vi "ADC Get Current Setup.vi"(8 "error in":errorcluster, 11 "adc session in":T12={"niScope"={"channel cfg"=[], "sessions"=[], "multi cards"=FALSE, "channels"=0, "type"=enum."n/a", "memory [B/chn]"=0, "ext. clock [Hz]"=0.0, "samples count"=0, "use streaming"=FALSE, "proc setup"={"packet size [smpl]"=0, "current timeout [s]"=0.0, "blk2blk timeout [s]"=0.0, "event time"=timestamp(0 s since 1904-01-01), "temp sampl T [s]"=0.0, "data queue"=refnum, "stop notifier"=refnum, "proc ref"=refnum}, "sample width [B]"=0, "ranges [V]"=[], "trigger setup"={"coupling"=1, "level [V]"=0.0, "slope"=0, "mode"=enum."Immediate"}, "fs [Hz]"=0.0, "bitres [bit]"=0}, "3458A"={"channels"=[], "sync unit"={"VISA"="", "type"=enum."Picotest U6200A"}, "awg unit"={"type"=enum."Agilent 331xxA to 332xxA", "VISA"="", "enable 10MHz ref"=FALSE}, "sync mode"=enum."MASTER-SLAVE, MASTER clocked by TIMER", "streaming mode"=FALSE, "idn mode"=enum."Auto", "sampling mode"=enum."DCV", "Ts [s]"=0.0, "sample memory [B]"=0, "proc setup"={"channel id"=0, "packet size [smpl]"=0, "current timeout [s]"=0.0, "blk2blk timeout [s]"=0.0, "event time"=timestamp(0 s since 1904-01-01), "stop notifier"=refnum, "data queues"=[], "proc refs"=[], "bus semaphore"=refnum}, "sample size [B]"=0, "sample count"=0, "aux data"={"channel id"=0, "valid?"=[], "gain [V]"=[], "timestamp [s]"=[], "Ts [s]"=0.0, "abs timestamp"=timestamp(0 s since 1904-01-01), "t [deg C]"=[]}, "ranges [V]"=[], "aperture [s]"=0.0, "LEVEL trigger"={"edge"=enum."POS", "level [V]"=0.0, "coupling"=enum."DC"}, "trigger mode"=enum."AUTO", "measure temp.?"=FALSE, "disp mesages"=[], "shared bus?"=FALSE, "disable display?"=FALSE, "aper mode"=enum."Manual", "aper rules"=[]}, "dsdll"={"dsdll"={"dsdll path"=path "", "dsdll handle"=[], "output devices"=[], "capture devices"=[]}, "channels"=0, "device id"=0, "channel idns"=[], "proc setup"={"packet size [smpl]"=0, "current timeout [s]"=0.0, "blk2blk timeout [s]"=0.0, "event time"=timestamp(0 s since 1904-01-01), "data queue"=refnum, "stop notifier"=refnum, "proc ref"=refnum}, "samples count"=0, "fs [Hz]"=0.0}, "type"=enum."niScope", "channel idn str"=[], "aux instr idn str"=[], "modified?"=FALSE, "simadc"={"channels"=[], "range [V]"=0.0, "Ts step [s]"=0.0, "time [s]"=0.0, "fs [Hz]"=0.0, "count"=0, "smpl offset"=0, "set count"=0, "bit res"=0}, "force rst?"=FALSE, "exit mode"=enum."Immediate reset", "exit dly"=0.0, "exit tmr"=timestamp(0 s since 1904-01-01), "busy?"=FALSE, "accessed?"=FALSE, "QuADC session"={"channel cfg"=[], "sessions"=[], "multi cards"=FALSE, "channels"=0, "type"=enum."n/a", "memory [B/chn]"=0, "ext. clock [Hz]"=0.0, "samples count"=0, "use streaming"=FALSE, "proc setup"={"packet size [smpl]"=0, "current timeout [s]"=0.0, "blk2blk timeout [s]"=0.0, "event time"=timestamp(0 s since 1904-01-01), "temp sampl T [s]"=0.0, "data queue"=refnum, "stop notifier"=refnum, "proc ref"=refnum}, "sample width [B]"=0, "ranges [V]"=[], "trigger setup"={"coupling"=1, "level [V]"=0.0, "slope"=0, "mode"=enum."Immediate"}, "fs [Hz]"=0.0, "bitres [bit]"=0}} {"QuADC session"."trigger setup"."level [V]" format="%.2f"; "QuADC session"."trigger setup"."coupling" items=["AC"=0, "DC"=1, "HF Reject"=3, "LF Reject"=4, "AC Plus HF Reject"=1001]; "QuADC session"."channel cfg"."Range [Vpk]" min=0.0; "QuADC session"."channel cfg"."Channel" min=0; "3458A"."channels"."Range [Vpk]" min=0.0; "niScope"."trigger setup"."level [V]" format="%.2f"; "niScope"."trigger setup"."coupling" items=["AC"=0, "DC"=1, "HF Reject"=3, "LF Reject"=4, "AC Plus HF Reject"=1001]; "niScope"."channel cfg"."Range [Vpk]" min=0.0; "niScope"."channel cfg"."Channel" min=0}) -> (0 "error out":errorcluster, 1 "device specific attributes":T9[](array[typedef]), 2 "common attributes":T4, 3 "adc session out":T12={"niScope"={"channel cfg"=[], "sessions"=[], "multi cards"=FALSE, "channels"=0, "type"=enum."n/a", "memory [B/chn]"=0, "ext. clock [Hz]"=0.0, "samples count"=0, "use streaming"=FALSE, "proc setup"={"packet size [smpl]"=0, "current timeout [s]"=0.0, "blk2blk timeout [s]"=0.0, "event time"=timestamp(0 s since 1904-01-01), "temp sampl T [s]"=0.0, "data queue"=refnum, "stop notifier"=refnum, "proc ref"=refnum}, "sample width [B]"=0, "ranges [V]"=[], "trigger setup"={"coupling"=1, "level [V]"=0.0, "slope"=0, "mode"=enum."Immediate"}, "fs [Hz]"=0.0, "bitres [bit]"=0}, "3458A"={"channels"=[], "sync unit"={"VISA"="", "type"=enum."Picotest U6200A"}, "awg unit"={"type"=enum."Agilent 331xxA to 332xxA", "VISA"="", "enable 10MHz ref"=FALSE}, "sync mode"=enum."MASTER-SLAVE, MASTER clocked by TIMER", "streaming mode"=FALSE, "idn mode"=enum."Auto", "sampling mode"=enum."DCV", "Ts [s]"=0.0, "sample memory [B]"=0, "proc setup"={"channel id"=0, "packet size [smpl]"=0, "current timeout [s]"=0.0, "blk2blk timeout [s]"=0.0, "event time"=timestamp(0 s since 1904-01-01), "stop notifier"=refnum, "data queues"=[], "proc refs"=[], "bus semaphore"=refnum}, "sample size [B]"=0, "sample count"=0, "aux data"={"channel id"=0, "valid?"=[], "gain [V]"=[], "timestamp [s]"=[], "Ts [s]"=0.0, "abs timestamp"=timestamp(0 s since 1904-01-01), "t [deg C]"=[]}, "ranges [V]"=[], "aperture [s]"=0.0, "LEVEL trigger"={"edge"=enum."POS", "level [V]"=0.0, "coupling"=enum."DC"}, "trigger mode"=enum."AUTO", "measure temp.?"=FALSE, "disp mesages"=[], "shared bus?"=FALSE, "disable display?"=FALSE, "aper mode"=enum."Manual", "aper rules"=[]}, "dsdll"={"dsdll"={"dsdll path"=path "", "dsdll handle"=[], "output devices"=[], "capture devices"=[]}, "channels"=0, "device id"=0, "channel idns"=[], "proc setup"={"packet size [smpl]"=0, "current timeout [s]"=0.0, "blk2blk timeout [s]"=0.0, "event time"=timestamp(0 s since 1904-01-01), "data queue"=refnum, "stop notifier"=refnum, "proc ref"=refnum}, "samples count"=0, "fs [Hz]"=0.0}, "type"=enum."niScope", "channel idn str"=[], "aux instr idn str"=[], "modified?"=FALSE, "simadc"={"channels"=[], "range [V]"=0.0, "Ts step [s]"=0.0, "time [s]"=0.0, "fs [Hz]"=0.0, "count"=0, "smpl offset"=0, "set count"=0, "bit res"=0}, "force rst?"=FALSE, "exit mode"=enum."Immediate reset", "exit dly"=0.0, "exit tmr"=timestamp(0 s since 1904-01-01), "busy?"=FALSE, "accessed?"=FALSE, "QuADC session"={"channel cfg"=[], "sessions"=[], "multi cards"=FALSE, "channels"=0, "type"=enum."n/a", "memory [B/chn]"=0, "ext. clock [Hz]"=0.0, "samples count"=0, "use streaming"=FALSE, "proc setup"={"packet size [smpl]"=0, "current timeout [s]"=0.0, "blk2blk timeout [s]"=0.0, "event time"=timestamp(0 s since 1904-01-01), "temp sampl T [s]"=0.0, "data queue"=refnum, "stop notifier"=refnum, "proc ref"=refnum}, "sample width [B]"=0, "ranges [V]"=[], "trigger setup"={"coupling"=1, "level [V]"=0.0, "slope"=0, "mode"=enum."Immediate"}, "fs [Hz]"=0.0, "bitres [bit]"=0}} {"QuADC session"."trigger setup"."level [V]" format="%.2f"; "QuADC session"."trigger setup"."coupling" items=["AC"=0, "DC"=1, "HF Reject"=3, "LF Reject"=4, "AC Plus HF Reject"=1001]; "QuADC session"."channel cfg"."Range [Vpk]" min=0.0; "QuADC session"."channel cfg"."Channel" min=0; "3458A"."channels"."Range [Vpk]" min=0.0; "niScope"."trigger setup"."level [V]" format="%.2f"; "niScope"."trigger setup"."coupling" items=["AC"=0, "DC"=1, "HF Reject"=3, "LF Reject"=4, "AC Plus HF Reject"=1001]; "niScope"."channel cfg"."Range [Vpk]" min=0.0; "niScope"."channel cfg"."Channel" min=0})   [LabVIEW 2013]
doc: "Returns current setup of the ADC (from session) so it will correctly work only after 'ADC Setup Virtual Channels'. It also returns device specific attributes as and array of names and text values."
uses:
  ADC Session.ctl
  drivers/niScope/niScope Session.ctl
  drivers/niScope/niScope Virtual Channel Config.ctl
  drivers/niScope/niScope Virtual Channel Mode.ctl
  drivers/niScope/niScope Virtual Channel Input Z.ctl
  drivers/niScope/niScope Virtual Channel Coupling.ctl
  drivers/niScope/niScope Type.ctl
  drivers/niScope/niScope Digitizing Process Options.ctl
  drivers/niScope/niScope Data Packet.ctl
  drivers/niScope/niScope Trigger Setup.ctl
  <instrlib>/niScope/Controls/niScope trigger coupling.ctl
  <instrlib>/niScope/Controls/niScope trigger slope.ctl
  drivers/DMM/3458A Digitizer Session.ctl
  drivers/DMM/3458A Virtual Channel Config.ctl
  drivers/Counter/Counter Session.ctl
  drivers/Counter/Counter Type.ctl
  drivers/AWG/AWG Session.ctl
  drivers/AWG/AWG Type.ctl
  drivers/DMM/3458A Sync Mode.ctl
  drivers/DMM/3458A Idn Mode.ctl
  drivers/DMM/3458A Digitizing Low Levels/Configure/Sampling Mode.ctl
  drivers/DMM/3458A Digitizing Process Options.ctl
  drivers/DMM/3458A Data Packet.ctl
  drivers/DMM/3458A Aux Record Data.ctl
  drivers/DMM/3458A Digitizing Low Levels/Configure/Level Setup.ctl
  drivers/DMM/3458A Digitizing Low Levels/Configure/First Sample Trigger.ctl
  drivers/DMM/3458A Aperture Selection Mode.ctl
  drivers/dsdll/DSDLL Session.ctl
  drivers/dsdll/dsdll.lvlibp/dsdll_instance.ctl
  drivers/dsdll/dsdll.lvlibp/dsdll_device_record.ctl
  drivers/dsdll/DSDLL Process Config.ctl
  drivers/dsdll/DSDLL Data Packet.ctl
  ADC Type.ctl
  drivers/simulated_adc/SimAdc Config.ctl
  drivers/simulated_adc/SimAdc Channel Cfg.ctl
  ADC On Close Action.ctl
  drivers/Quatsch_driver/QuADCDriver/QuADC Session.ctl
  drivers/Quatsch_driver/QuADCDriver/QuADC Virtual Channel Config.ctl
  drivers/Quatsch_driver/QuADCDriver/QuADC Virtual Channel Mode.ctl
  drivers/Quatsch_driver/QuADCDriver/QuADC Virtual Channel Input Z.ctl
  drivers/Quatsch_driver/QuADCDriver/QuADC Virtual Channel Coupling.ctl
  drivers/Quatsch_driver/QuADCDriver/QuADC Type.ctl
  drivers/Quatsch_driver/QuADCDriver/QuADC Digitizing Process Options.ctl
  drivers/Quatsch_driver/QuADCDriver/QuADC Data Packet.ctl
  drivers/Quatsch_driver/QuADCDriver/QuADC Trigger Setup.ctl
  ADC Attribute.ctl
  ADC Current Configuration.ctl
  ADC Trig Config.ctl
  ADC Trig Mode Source.ctl
  ADC Trig Coupling.ctl
  ADC Trig Slope.ctl
  drivers/DMM/3458A Virtual Digitizer.lvlib
  drivers/niScope/niScope Virtual Digitizer.lvlib
  drivers/Counter/Counter.lvlib
  drivers/AWG/AWG.lvlib
  drivers/DMM/3458A Digitizing Low Levels/3458A Digitizing Low Levels.lvlib
  drivers/dsdll/dsdll.lvlibp
  drivers/dsdll/DSDLL Virtual Digitizer.lvlib
  drivers/Quatsch_driver/QuADCDriver/QuADC Virtual Digitizer.lvlib
panel:
  in  "Coupling":T1=enum."DC"
  in  "Input Z":T2
  in  "Mode":T3
  in  "3458A.sync mode":T10
  in  "3458A.sampling mode":T11
  # "IP Address"
  # "."
  # "."
  # "."
  # ":"
  # "IP Address"
  # "."
  # "."
  # "."
  # ":"
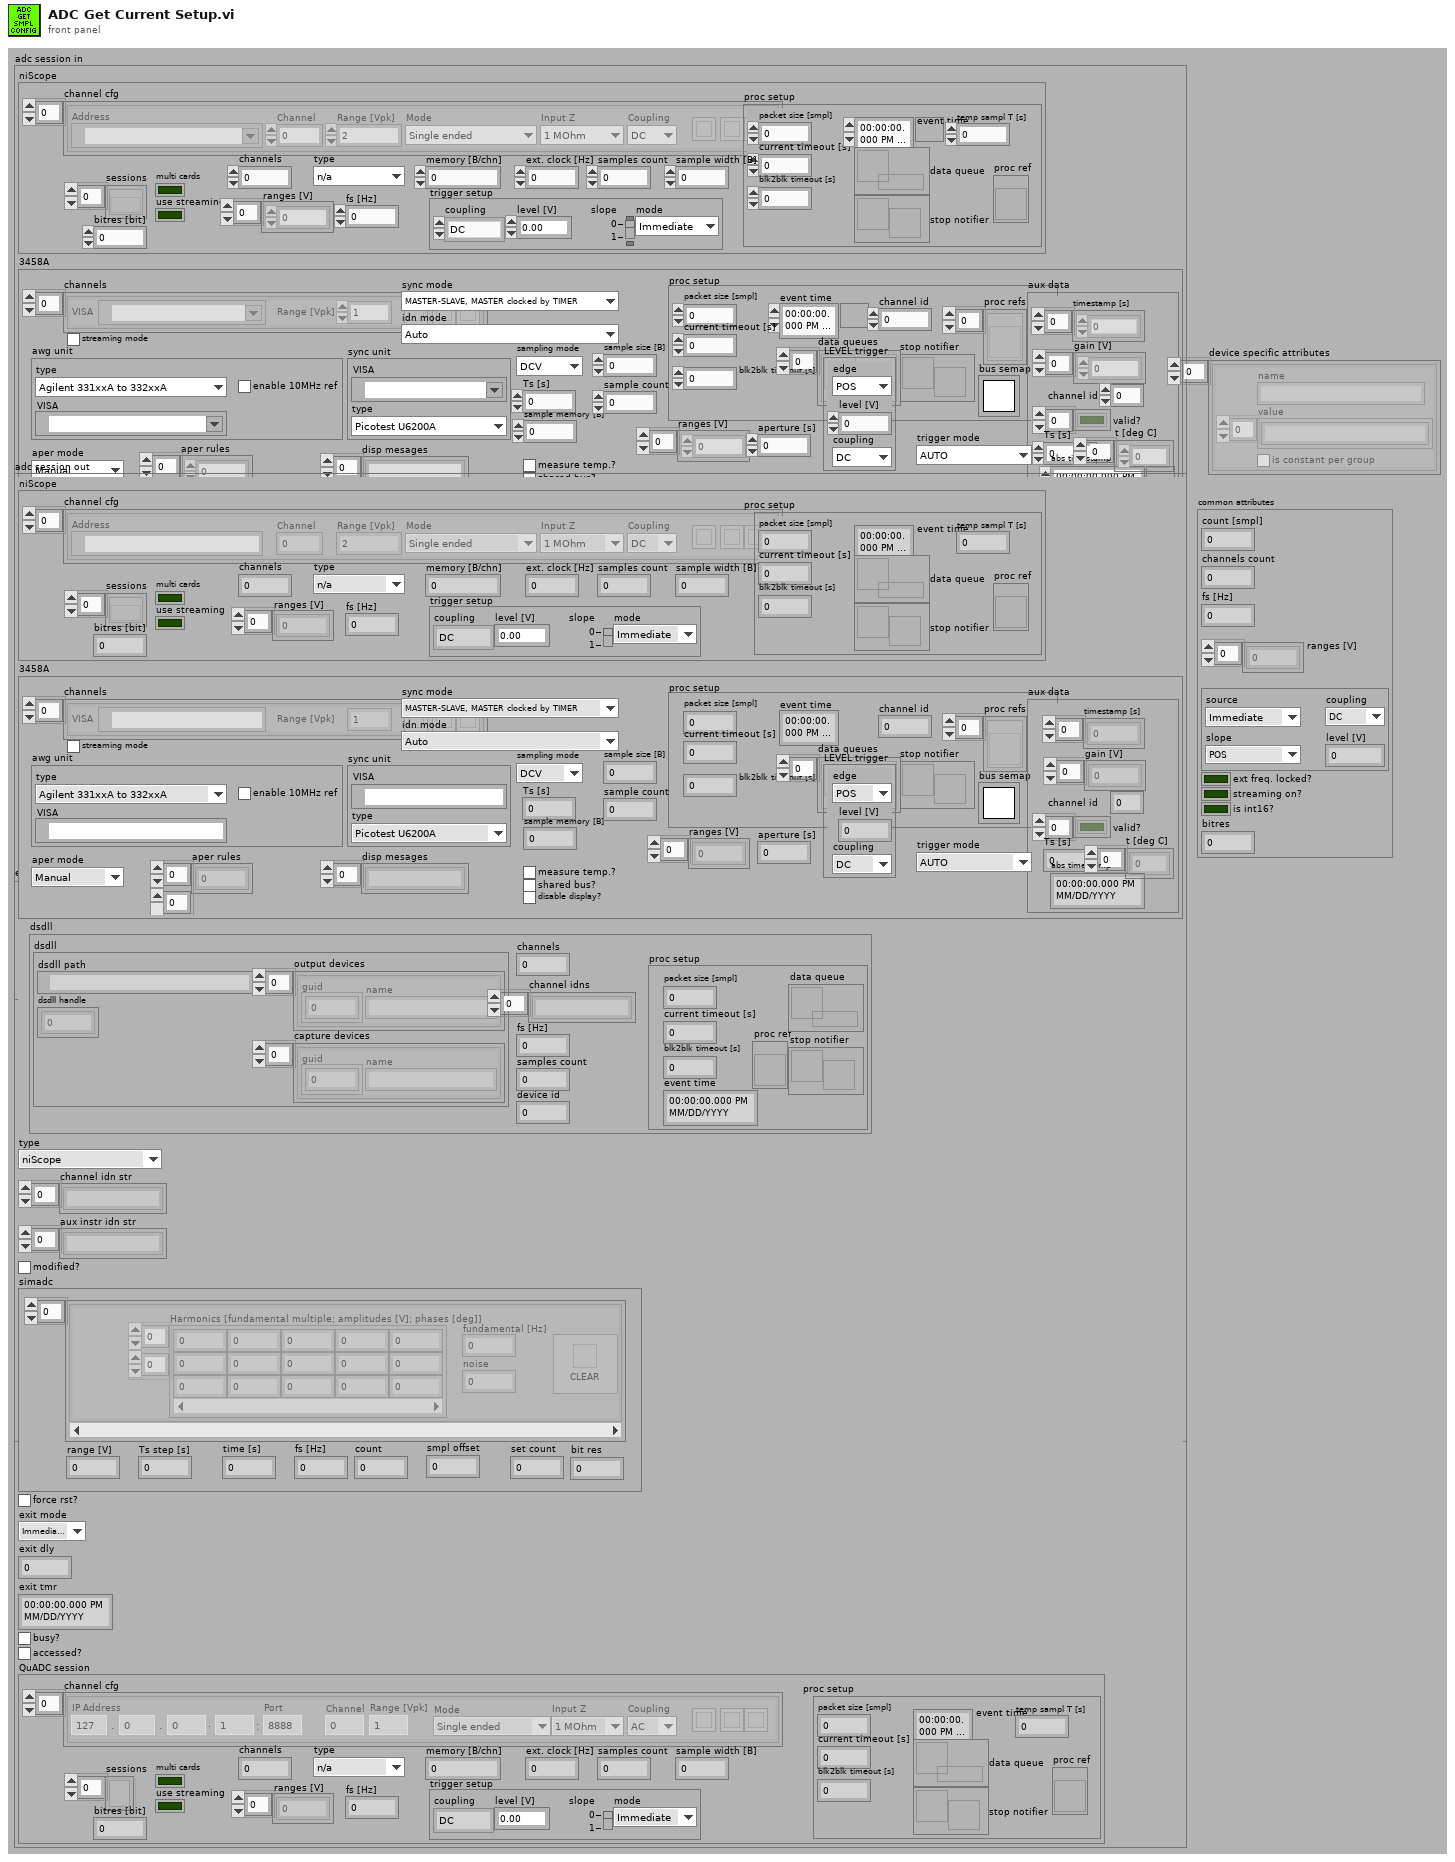
[diagram p1: front panel]
types:
  T1 = typedef "niScope Virtual Digitizer.lvlib/niScope Virtual Channel Coupling.ctl" = enum16{"AC", "DC", "GND"}
  T2 = typedef "niScope Virtual Digitizer.lvlib/niScope Virtual Channel Input Z.ctl" = enum16{"1 MOhm", "50 Ohm"}
  T3 = typedef "niScope Virtual Digitizer.lvlib/niScope Virtual Channel Mode.ctl" = enum16{"Single ended", "Unbal. differential", "Differential"}
  T4 = typedef "ADC Current Configuration.ctl" = cluster{"count [smpl]":i64, "channels count":i32, "fs [Hz]":dbl, "ranges [V]":dbl[], "trigger":T5, "ext freq. locked?":bool, "streaming on?":bool, "is int16?":bool, "bitres":i32}
  T5 = typedef "ADC Trig Config.ctl" = cluster{"source":T6, "level [V]":dbl, "coupling":T7, "slope":T8}
  T6 = typedef "ADC Trig Mode Source.ctl" = enum16{"Immediate", "External", "Level"}
  T7 = typedef "ADC Trig Coupling.ctl" = enum16{"DC", "AC"}
  T8 = typedef "ADC Trig Slope.ctl" = enum16{"POS", "NEG"}
  T9 = typedef "ADC Attribute.ctl" = cluster{"name":string, "value":string[], "is constant per group":bool}
  T10 = typedef "3458A Virtual Digitizer.lvlib/3458A Sync Mode.ctl" = enum16{"MASTER-SLAVE, MASTER clocked by TIMER", "MASTER-SLAVE, MASTER clocked by AWG", "ALL clocked by AWG", "MASTER-SLAVE, ALL clocked by TIMER", "ALL clocked by AWG with DFLL"}
  T11 = typedef "3458A Virtual Digitizer.lvlib/3458A Digitizing Low Levels.lvlib/Sampling Mode.ctl" = enum16{"DCV", "DSDC", "DSAC"}
  T12 = typedef "ADC Session.ctl" = cluster{"niScope":T13, "3458A":T20, "dsdll":T33, "type":T37, "channel idn str":string[], "aux instr idn str":string[], "modified?":bool, "simadc":T38, "force rst?":bool, "exit mode":T40, "exit dly":dbl, "exit tmr":timestamp, "busy?":bool, "accessed?":bool, "QuADC session":T41}
  T13 = typedef "niScope Virtual Digitizer.lvlib/niScope Session.ctl" = cluster{"channel cfg":T14[], "sessions":refnum<k20>[], "multi cards":bool, "channels":i32, "type":T15, "memory [B/chn]":i32, "ext. clock [Hz]":dbl, "samples count":i64, "use streaming":bool, "proc setup":T16, "sample width [B]":i32, "ranges [V]":dbl[], "trigger setup":T17, "fs [Hz]":dbl, "bitres [bit]":i32}
  T14 = typedef "niScope Virtual Digitizer.lvlib/niScope Virtual Channel Config.ctl" = cluster{"Address":refnum<k15>, "Channel":i32, "Mode":T3, "Input Z":T2, "Coupling":T1, "Range [Vpk]":dbl, "btn clr":bool, "btn up":bool, "btn down":bool}
  T15 = typedef "niScope Virtual Digitizer.lvlib/niScope Type.ctl" = enum16{"n/a", "5922"}
  T16 = typedef "niScope Virtual Digitizer.lvlib/niScope Digitizing Process Options.ctl" = cluster{"packet size [smpl]":i64, "current timeout [s]":dbl, "blk2blk timeout [s]":dbl, "event time":timestamp, "temp sampl T [s]":dbl, "data queue":refnum<queue>, "stop notifier":refnum<notifier>, "proc ref":refnum<vi>}
  T17 = typedef "niScope Virtual Digitizer.lvlib/niScope Trigger Setup.ctl" = cluster{"coupling":T18, "level [V]":dbl, "slope":T19, "mode":enum16{"Immediate", "External", "Level"}}
  T18 = typedef "niScope trigger coupling.ctl" = u16
  T19 = typedef "niScope trigger slope.ctl" = i32
  T20 = typedef "3458A Virtual Digitizer.lvlib/3458A Digitizer Session.ctl" = cluster{"channels":T21[], "sync unit":T22, "awg unit":T24, "sync mode":T10, "streaming mode":bool, "idn mode":T26, "sampling mode":T11, "Ts [s]":dbl, "sample memory [B]":i32, "proc setup":T27, "sample size [B]":i32, "sample count":i32, "aux data":T29, "ranges [V]":dbl[], "aperture [s]":dbl, "LEVEL trigger":T30, "trigger mode":T31, "measure temp.?":bool, "disp mesages":string[], "shared bus?":bool, "disable display?":bool, "aper mode":T32, "aper rules":dbl[][]}
  T21 = typedef "3458A Virtual Digitizer.lvlib/3458A Virtual Channel Config.ctl" = cluster{"VISA":refnum<visa-resource-name>, "Range [Vpk]":dbl, "btn clr":bool, "btn up":bool, "btn down":bool}
  T22 = typedef "Counter.lvlib/Counter Session.ctl" = cluster{"VISA":refnum<visa-resource-name>, "type":T23}
  T23 = typedef "Counter.lvlib/Counter Type.ctl" = enum16{"Picotest U6200A", "dummy"}
  T24 = typedef "AWG.lvlib/AWG Session.ctl" = cluster{"type":T25, "VISA":refnum<visa-resource-name>, "enable 10MHz ref":bool}
  T25 = typedef "AWG.lvlib/AWG Type.ctl" = enum16{"Agilent 331xxA to 332xxA", "Agilent 335xxA to 336xxA", "Tektronix AFG3101C", "dummy"}
  T26 = typedef "3458A Virtual Digitizer.lvlib/3458A Idn Mode.ctl" = enum16{"Auto", "Sequential (chn A, chn B, ...)", "From calibration string"}
  T27 = typedef "3458A Virtual Digitizer.lvlib/3458A Digitizing Process Options.ctl" = cluster{"channel id":i32, "packet size [smpl]":i32, "current timeout [s]":dbl, "blk2blk timeout [s]":dbl, "event time":timestamp, "stop notifier":refnum<notifier>, "data queues":refnum<queue>[], "proc refs":refnum<vi>[], "bus semaphore":T28}
  T28 = typedef "Semaphore RefNum" = refnum<k1>
  T29 = typedef "3458A Virtual Digitizer.lvlib/3458A Aux Record Data.ctl" = cluster{"channel id":i32, "valid?":bool[], "gain [V]":dbl[], "timestamp [s]":dbl[], "Ts [s]":dbl, "abs timestamp":timestamp, "t [deg C]":dbl[]}
  T30 = typedef "3458A Virtual Digitizer.lvlib/3458A Digitizing Low Levels.lvlib/Level Setup.ctl" = cluster{"edge":enum16{"POS", "NEG"}, "level [V]":dbl, "coupling":enum16{"DC", "AC"}}
  T31 = typedef "3458A Virtual Digitizer.lvlib/3458A Digitizing Low Levels.lvlib/First Sample Trigger.ctl" = enum16{"AUTO", "EXT", "SYN", "SGL", "HOLD", "LEVEL"}
  T32 = typedef "3458A Virtual Digitizer.lvlib/3458A Aperture Selection Mode.ctl" = enum16{"Manual", "Maximum", "Table"}
  T33 = typedef "DSDLL Virtual Digitizer.lvlib/DSDLL Session.ctl" = cluster{"dsdll":T34, "channels":i32, "device id":i32, "channel idns":string[], "proc setup":T36, "samples count":i32, "fs [Hz]":dbl}
  T34 = typedef "dsdll.lvlibp/dsdll_instance.ctl" = cluster{"dsdll path":path, "dsdll handle":u8[], "output devices":T35[], "capture devices":T35[]}
  T35 = typedef "dsdll.lvlibp/dsdll_device_record.ctl" = cluster{"guid":u8[], "name":string}
  T36 = typedef "DSDLL Virtual Digitizer.lvlib/DSDLL Process Config.ctl" = cluster{"packet size [smpl]":i32, "current timeout [s]":dbl, "blk2blk timeout [s]":dbl, "event time":timestamp, "data queue":refnum<queue>, "stop notifier":refnum<notifier>, "proc ref":refnum<vi>}
  T37 = typedef "ADC Type.ctl" = enum16{"niScope", "3458A", "DirectSound DLL", "dummy", "QuADC"}
  T38 = typedef "SimAdc Config.ctl" = cluster{"channels":T39[], "range [V]":dbl, "Ts step [s]":dbl, "time [s]":dbl, "fs [Hz]":dbl, "count":i64, "smpl offset":i64, "set count":i64, "bit res":i32}
  T39 = typedef "SimAdc Channel Cfg.ctl" = cluster{"harmonics":dbl[][], "btn clear":bool, "noise":dbl, "fundamental [Hz]":dbl}
  T40 = typedef "ADC On Close Action.ctl" = enum16{"Immediate reset", "Delayed reset"}
  T41 = typedef "QuADC Virtual Digitizer.lvlib/QuADC Session.ctl" = cluster{"channel cfg":T42[], "sessions":refnum<k5>[], "multi cards":bool, "channels":i32, "type":T46, "memory [B/chn]":i32, "ext. clock [Hz]":dbl, "samples count":i64, "use streaming":bool, "proc setup":T47, "sample width [B]":i32, "ranges [V]":dbl[], "trigger setup":T48, "fs [Hz]":dbl, "bitres [bit]":i32}
  T42 = typedef "QuADC Virtual Digitizer.lvlib/QuADC Virtual Channel Config.ctl" = cluster{"Channel":i32, "Mode":T43, "Input Z":T44, "Coupling":T45, "Range [Vpk]":dbl, "btn clr":bool, "btn up":bool, "btn down":bool, "IP address A":u8, "IP address B":u8, "IP address C":u8, "IP address D":u8, "Port":u16}
  T43 = typedef "QuADC Virtual Digitizer.lvlib/QuADC Virtual Channel Mode.ctl" = enum16{"Single ended", "Unbal. differential", "Differential"}
  T44 = typedef "QuADC Virtual Digitizer.lvlib/QuADC Virtual Channel Input Z.ctl" = enum16{"1 MOhm", "50 Ohm"}
  T45 = typedef "QuADC Virtual Digitizer.lvlib/QuADC Virtual Channel Coupling.ctl" = enum16{"AC", "DC", "GND"}
  T46 = typedef "QuADC Virtual Digitizer.lvlib/QuADC Type.ctl" = enum16{"n/a", "v1"}
  T47 = typedef "QuADC Virtual Digitizer.lvlib/QuADC Digitizing Process Options.ctl" = cluster{"packet size [smpl]":i64, "current timeout [s]":dbl, "blk2blk timeout [s]":dbl, "event time":timestamp, "temp sampl T [s]":dbl, "data queue":refnum<queue>, "stop notifier":refnum<notifier>, "proc ref":refnum<vi>}
  T48 = typedef "QuADC Virtual Digitizer.lvlib/QuADC Trigger Setup.ctl" = cluster{"coupling":T18, "level [V]":dbl, "slope":T19, "mode":enum16{"Immediate", "External", "Level"}}
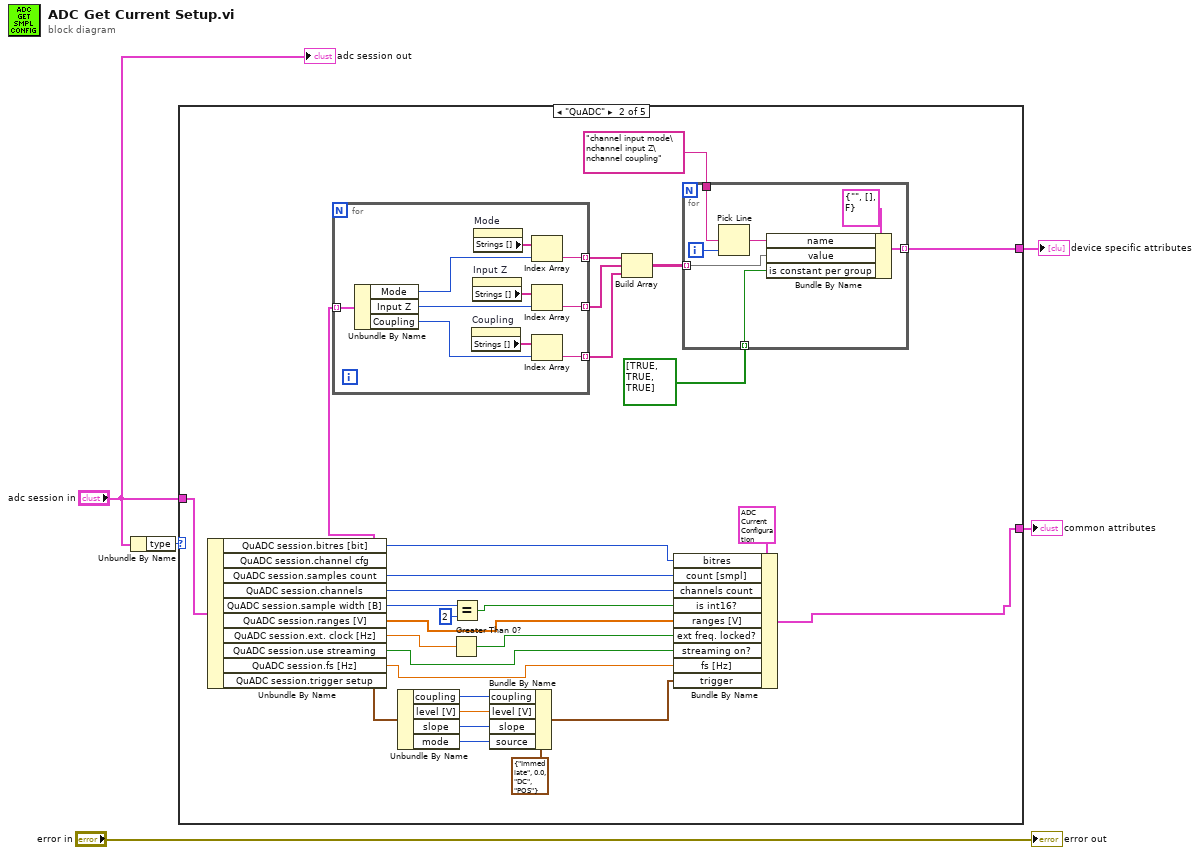
[diagram p0: block diagram]
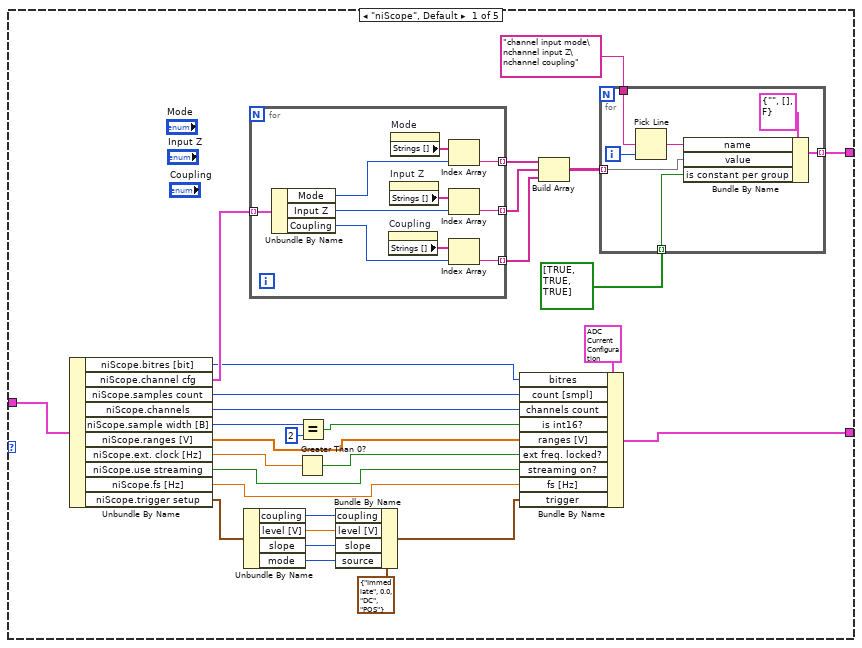
[diagram p2: hidden frame]
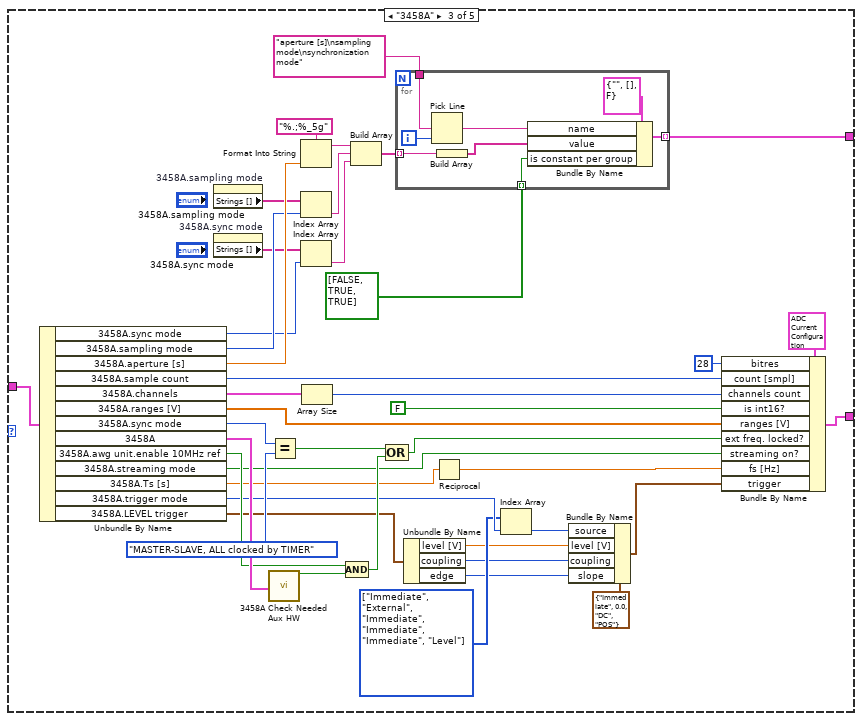
[diagram p3: hidden frame]
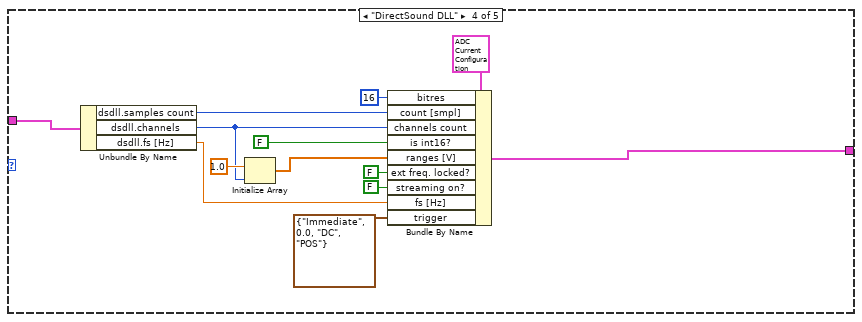
[diagram p4: hidden frame]
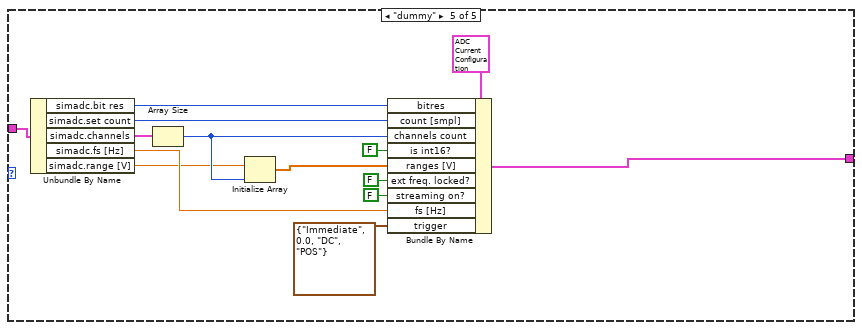
[diagram p5: hidden frame]
diagram:
  n1 = Unbundle By Name("adc session in") -> ("type"=w5:T37)
  n2 = case shown="\"QuADC\"" w5 {
    tunnel: "adc session in" -> [w34 w55 w139 w160 w174]
    tunnel: [w8 w53 w126 _ _] -> w2
    tunnel: [w23 w54 w112 w151 w167] -> w1
    frame "niScope", Default {
      n3 = Unbundle By Name(w34) -> ("niScope.bitres [bit]"=w7:i32, "niScope.channel cfg"=w14:T14[], "niScope.samples count"=w30:i64, "niScope.channels"=w29:i32, "niScope.sample width [B]"=w33:i32, "niScope.ranges [V]"=w27:dbl[], "niScope.ext. clock [Hz]"=w26:dbl, "niScope.use streaming"=w24:bool, "niScope.fs [Hz]"=w22:dbl, "niScope.trigger setup"=w21:T17)
      n4 = Unbundle By Name(w21) -> ("coupling"=w19:T18, "level [V]"=w18:dbl, "slope"=w17:T19, "mode"=w16:enum16{"Immediate", "External", "Level"})
      n5 = for {
        tunnel: w14 -> [w51] mode=indexing
        tunnel: [w48] -> w12 mode=indexing
        tunnel: [w45] -> w11 mode=indexing
        tunnel: [w42] -> w10 mode=indexing
        n6 = Unbundle By Name(w51) -> ("Mode"=w50:T3, "Input Z"=w46:T2, "Coupling"=w43:T1)
        n7 = property on="Coupling" class="Enum (strict)"() -> ("Strings []"=w44:string[])  [unwired: 2 in, 2 out]
        n8 = property on="Input Z" class="Enum (strict)"() -> ("Strings []"=w47:string[])  [unwired: 2 in, 2 out]
        n9 = property on="Mode" class="Enum (strict)"() -> ("Strings []"=w49:string[])  [unwired: 2 in, 2 out]
        n10 = Index Array(array=w49, index=w50) -> (element=w48:string)
        n11 = Index Array(array=w47, index=w46) -> (element=w45:string)
        n12 = Index Array(array=w44, index=w43) -> (element=w42:string)
      }
      n13 = Greater Than 0?(x=w26) -> (x > 0?=w25:bool)
      n14 = Equal?(x=w33, y=2) -> (x = y?=w28:bool)
      n15 = Bundle By Name(cluster=T5 {"source"=enum."Immediate", "level [V]"=0.0, "coupling"=enum."DC", "slope"=enum."POS"} ("trigger"), "coupling"=w19, "level [V]"=w18, "slope"=w17, "source"=w16) -> (w15:T5)
      n16 = Bundle By Name(cluster=T4 {"count [smpl]"=0, "channels count"=0, "fs [Hz]"=0.0, "ranges [V]"=[], "trigger"={"source"=enum."Immediate", "level [V]"=0.0, "coupling"=enum."DC", "slope"=enum."POS"}, "ext freq. locked?"=FALSE, "streaming on?"=FALSE, "is int16?"=FALSE, "bitres"=0} ("common attributes"), "bitres"=w7, "count [smpl]"=w30, "channels count"=w29, "is int16?"=w28, "ranges [V]"=w27, "ext freq. locked?"=w25, "streaming on?"=w24, "fs [Hz]"=w22, "trigger"=w15) -> (w23:T4)
      n17 = Build Array(w12, w11, w10) -> (w9:string[][])
      n18 = for {
        tunnel: "channel input mode\nchannel input Z\nchannel coupling" -> [w40]
        tunnel: [w37] -> w8 mode=indexing
        tunnel: w9 -> [w36] mode=indexing
        tunnel: bool[] [TRUE, TRUE, TRUE] -> [w35] mode=indexing
        i -> [w39]
        n19 = Pick Line(multi-line string=w40, line index=w39) -> (output string=w38:string)  [unwired: 1 in]
        n20 = Bundle By Name(cluster=T9 {"name"="", "value"=[], "is constant per group"=FALSE} ("adc attribute"), "name"=w38, "value"=w36, "is constant per group"=w35) -> (w37:T9)
      }
    }
    frame "QuADC" {
      n21 = Unbundle By Name(w55) -> ("QuADC session.bitres [bit]"=w56:i32, "QuADC session.channel cfg"=w52:T42[], "QuADC session.samples count"=w71:i64, "QuADC session.channels"=w70:i32, "QuADC session.sample width [B]"=w74:i32, "QuADC session.ranges [V]"=w68:dbl[], "QuADC session.ext. clock [Hz]"=w67:dbl, "QuADC session.use streaming"=w65:bool, "QuADC session.fs [Hz]"=w64:dbl, "QuADC session.trigger setup"=w63:T48)
      n22 = for {
        tunnel: w52 -> [w97] mode=indexing
        tunnel: [w94] -> w79 mode=indexing
        tunnel: [w91] -> w78 mode=indexing
        tunnel: [w88] -> w77 mode=indexing
        n23 = Unbundle By Name(w97) -> ("Mode"=w96:T43, "Input Z"=w92:T44, "Coupling"=w89:T45)
        n24 = property on="Coupling" class="Enum (strict)"() -> ("Strings []"=w90:string[])  [unwired: 2 in, 2 out]
        n25 = property on="Input Z" class="Enum (strict)"() -> ("Strings []"=w93:string[])  [unwired: 2 in, 2 out]
        n26 = property on="Mode" class="Enum (strict)"() -> ("Strings []"=w95:string[])  [unwired: 2 in, 2 out]
        n27 = Index Array(array=w95, index=w96) -> (element=w94:string)
        n28 = Index Array(array=w93, index=w92) -> (element=w91:string)
        n29 = Index Array(array=w90, index=w89) -> (element=w88:string)
      }
      n30 = Unbundle By Name(w63) -> ("coupling"=w61:T18, "level [V]"=w60:dbl, "slope"=w59:T19, "mode"=w58:enum16{"Immediate", "External", "Level"})
      n31 = Greater Than 0?(x=w67) -> (x > 0?=w66:bool)
      n32 = Equal?(x=w74, y=2) -> (x = y?=w69:bool)
      n33 = Bundle By Name(cluster=T5 {"source"=enum."Immediate", "level [V]"=0.0, "coupling"=enum."DC", "slope"=enum."POS"} ("trigger"), "coupling"=w61, "level [V]"=w60, "slope"=w59, "source"=w58) -> (w57:T5)
      n34 = Build Array(w79, w78, w77) -> (w76:string[][])
      n35 = Bundle By Name(cluster=T4 {"count [smpl]"=0, "channels count"=0, "fs [Hz]"=0.0, "ranges [V]"=[], "trigger"={"source"=enum."Immediate", "level [V]"=0.0, "coupling"=enum."DC", "slope"=enum."POS"}, "ext freq. locked?"=FALSE, "streaming on?"=FALSE, "is int16?"=FALSE, "bitres"=0} ("common attributes"), "bitres"=w56, "count [smpl]"=w71, "channels count"=w70, "is int16?"=w69, "ranges [V]"=w68, "ext freq. locked?"=w66, "streaming on?"=w65, "fs [Hz]"=w64, "trigger"=w57) -> (w54:T4)
      n36 = for {
        tunnel: "channel input mode\nchannel input Z\nchannel coupling" -> [w86]
        tunnel: [w83] -> w53 mode=indexing
        tunnel: w76 -> [w82] mode=indexing
        tunnel: bool[] [TRUE, TRUE, TRUE] -> [w81] mode=indexing
        i -> [w85]
        n37 = Pick Line(multi-line string=w86, line index=w85) -> (output string=w84:string)  [unwired: 1 in]
        n38 = Bundle By Name(cluster=T9 {"name"="", "value"=[], "is constant per group"=FALSE} ("adc attribute"), "name"=w84, "value"=w82, "is constant per group"=w81) -> (w83:T9)
      }
    }
    frame "3458A" {
      w106 = T6[] [enum."Immediate", enum."External", enum."Immediate", enum."Immediate", enum."Immediate", enum."Level"] items=["Immediate", "External", "Level"]
      n39 = Unbundle By Name(w139) -> ("3458A.sync mode"=w132:T10, "3458A.sampling mode"=w134:T11, "3458A.aperture [s]"=w136:dbl, "3458A.sample count"=w124:i32, "3458A.channels"=w138:T21[], "3458A.ranges [V]"=w122:dbl[], "3458A.sync mode"=w121:T10, "3458A"=w117:T20, "3458A.awg unit.enable 10MHz ref"=w116:bool, "3458A.streaming mode"=w113:bool, "3458A.Ts [s]"=w110:dbl, "3458A.trigger mode"=w107:T31, "3458A.LEVEL trigger"=w104:T30)
      n40 = property on="3458A.sampling mode" class="Enum (strict)"() -> ("Strings []"=w135:string[])  [unwired: 2 in, 2 out]
      n41 = property on="3458A.sync mode" class="Enum (strict)"() -> ("Strings []"=w133:string[])  [unwired: 2 in, 2 out]
      n42 = call "3458A Check Needed Aux HW.vi"("digitizer session"=w117) -> ("uses AWG clocking?"=w115:bool)  [unwired: 13 in, 5 out]
      n43 = Equal?(x=w121, y=3458A_Sync_Mode."MASTER-SLAVE, ALL clocked by TIMER") -> (x = y?=w119:bool)
      n44 = Format Into String(format string="%.;%_5g", w136) -> (resulting string=w130:string)  [unwired: 2 in, 1 out]
      n45 = Index Array(array=w135, index=w134) -> (element=w129:string)
      n46 = Index Array(array=w133, index=w132) -> (element=w128:string)
      n47 = Array Size(array=w138) -> (size(s)=w100:i32)
      n48 = Compound Arithmetic op=AND(w116, w115) -> (w114:bool)
      n49 = Build Array(w130, w129, w128) -> (w127:string[])
      n50 = Compound Arithmetic op=OR(w119, w114) -> (w118:bool)
      n51 = for {
        tunnel: "aperture [s]\nsampling mode\nsynchronization mode" -> [w146]
        tunnel: [w143] -> w126 mode=indexing
        tunnel: w127 -> [w142] mode=indexing
        tunnel: bool[] [FALSE, TRUE, TRUE] -> [w140] mode=indexing
        i -> [w145]
        n52 = Pick Line(multi-line string=w146, line index=w145) -> (output string=w144:string)  [unwired: 1 in]
        n53 = Build Array(w142) -> (w141:string[])
        n54 = Bundle By Name(cluster=T9 {"name"="", "value"=[], "is constant per group"=FALSE} ("adc attribute"), "name"=w144, "value"=w141, "is constant per group"=w140) -> (w143:T9)
      }
      n55 = Unbundle By Name(w104) -> ("level [V]"=w103:dbl, "coupling"=w102:enum16{"DC", "AC"}, "edge"=w101:enum16{"POS", "NEG"})
      n56 = Reciprocal(x=w110) -> (1/x=w111:dbl)
      n57 = Index Array(array=w106, index=w107) -> (element=w105:T6)
      n58 = Bundle By Name(cluster=T5 {"source"=enum."Immediate", "level [V]"=0.0, "coupling"=enum."DC", "slope"=enum."POS"} ("trigger"), "source"=w105, "level [V]"=w103, "coupling"=w102, "slope"=w101) -> (w108:T5)
      n59 = Bundle By Name(cluster=T4 {"count [smpl]"=0, "channels count"=0, "fs [Hz]"=0.0, "ranges [V]"=[], "trigger"={"source"=enum."Immediate", "level [V]"=0.0, "coupling"=enum."DC", "slope"=enum."POS"}, "ext freq. locked?"=FALSE, "streaming on?"=FALSE, "is int16?"=FALSE, "bitres"=0} ("common attributes"), "bitres"=28, "count [smpl]"=w124, "channels count"=w100, "is int16?"=FALSE, "ranges [V]"=w122, "ext freq. locked?"=w118, "streaming on?"=w113, "fs [Hz]"=w111, "trigger"=w108) -> (w112:T4)
    }
    frame "DirectSound DLL" {
      n60 = Unbundle By Name(w160) -> ("dsdll.samples count"=w157:i32, "dsdll.channels"=w156:i32, "dsdll.fs [Hz]"=w150:dbl)
      n61 = Initialize Array(1.0 ("element"), w156) -> (w154:dbl[])
      n62 = Bundle By Name(cluster=T4 {"count [smpl]"=0, "channels count"=0, "fs [Hz]"=0.0, "ranges [V]"=[], "trigger"={"source"=enum."Immediate", "level [V]"=0.0, "coupling"=enum."DC", "slope"=enum."POS"}, "ext freq. locked?"=FALSE, "streaming on?"=FALSE, "is int16?"=FALSE, "bitres"=0} ("common attributes"), "bitres"=16, "count [smpl]"=w157, "channels count"=w156, "is int16?"=FALSE, "ranges [V]"=w154, "ext freq. locked?"=FALSE, "streaming on?"=FALSE, "fs [Hz]"=w150, "trigger"=T5 {"source"=enum."Immediate", "level [V]"=0.0, "coupling"=enum."DC", "slope"=enum."POS"}) -> (w151:T4)
    }
    frame "dummy" {
      n63 = Unbundle By Name(w174) -> ("simadc.bit res"=w161:i32, "simadc.set count"=w172:i64, "simadc.channels"=w164:T39[], "simadc.fs [Hz]"=w166:dbl, "simadc.range [V]"=w162:dbl)
      n64 = Array Size(array=w164) -> (size(s)=w163:i32)
      n65 = Initialize Array(w162, w163) -> (w170:dbl[])
      n66 = Bundle By Name(cluster=T4 {"count [smpl]"=0, "channels count"=0, "fs [Hz]"=0.0, "ranges [V]"=[], "trigger"={"source"=enum."Immediate", "level [V]"=0.0, "coupling"=enum."DC", "slope"=enum."POS"}, "ext freq. locked?"=FALSE, "streaming on?"=FALSE, "is int16?"=FALSE, "bitres"=0} ("common attributes"), "bitres"=w161, "count [smpl]"=w172, "channels count"=w163, "is int16?"=FALSE, "ranges [V]"=w170, "ext freq. locked?"=FALSE, "streaming on?"=FALSE, "fs [Hz]"=w166, "trigger"=T5 {"source"=enum."Immediate", "level [V]"=0.0, "coupling"=enum."DC", "slope"=enum."POS"}) -> (w167:T4)
    }
  }
  "device specific attributes" <- w2
  "common attributes" <- w1
  "error out" <- "error in"
  "adc session out" <- "adc session in"
